vi "generate_multiharm_signal_points.vi"(1 "Harmonics":T1(array[cluster]), 2 "Points Count":i32=1000000, 3 "Fout":dbl=1000000.0) -> (0 "Signal Points":dbl[](array[numeric]))   [LabVIEW 2010]
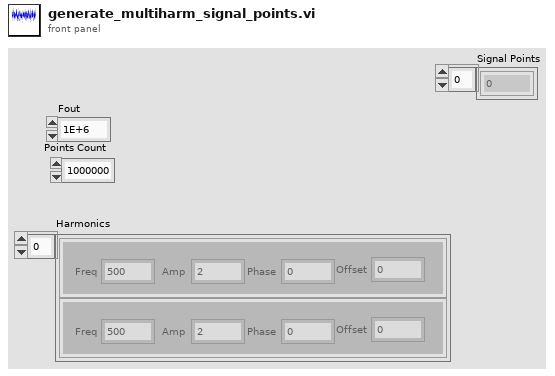
[diagram p1: front panel]
types:
  T1 = cluster{"Freq":dbl, "Amp":dbl, "Phase":dbl, "Offset":dbl}[]
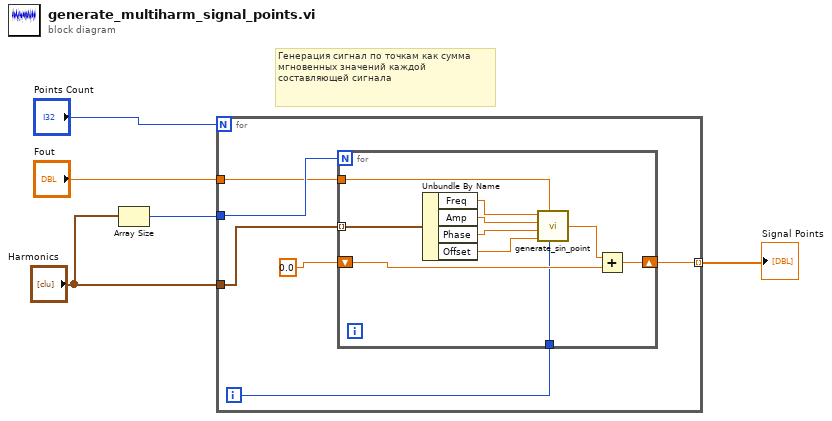
[diagram p0: block diagram]
diagram:
  # "Генерация сигнал по точкам как сумма мгновенных значений каждой составляющей сигнала"
  n1 = Array Size(array="Harmonics") -> (size(s)=w4:i32)
  n2 = for {
    N: "Points Count" -> [_]
    tunnel: w4 -> [w11]
    tunnel: "Harmonics" -> [w10]
    tunnel: "Fout" -> [w9]
    tunnel: [w7] -> w1 mode=indexing
    i -> [w6]
    n3 = for {
      N: w11 -> [_]
      tunnel: w10 -> [w21] mode=indexing
      tunnel: w9 -> [w16]
      shift-right: [w13] -> w7
      shift-left: 0.0 -> [w15]
      tunnel: w6 -> [w12]
      n4 = Unbundle By Name(w21) -> ("Freq"=w20:dbl, "Amp"=w19:dbl, "Phase"=w18:dbl, "Offset"=w17:dbl)
      n5 = call "generate_sin_point.vi"("Point Index"=w12, "Fout"=w16, "Offset"=w17, "Phase"=w18, "Amp"=w19, "Freq"=w20) -> ("Point Value"=w14:dbl)
      n6 = Add(x=w14, y=w15) -> (x+y=w13:dbl)
    }
  }
  "Signal Points" <- w1
